vi "sub_psk_symbol_map_gen.vi"(9 "Gray code?":bool=TRUE, 11 "M-PSK":i32=4) -> (1 "index map":u32[](array[numeric]), 3 "symbol map":cdb[](array[numeric]))   [LabVIEW 2014]
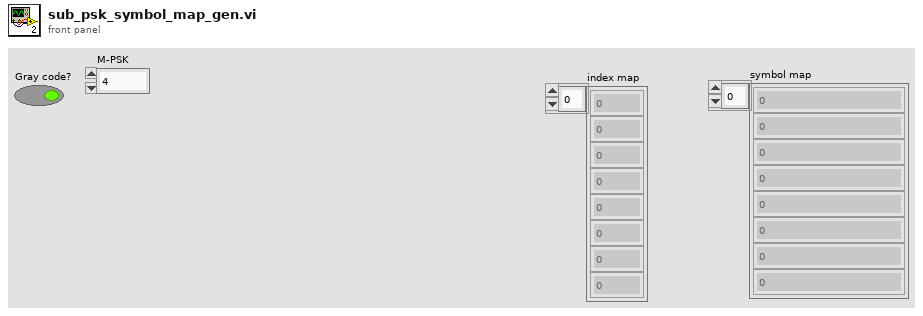
[diagram p1: front panel]
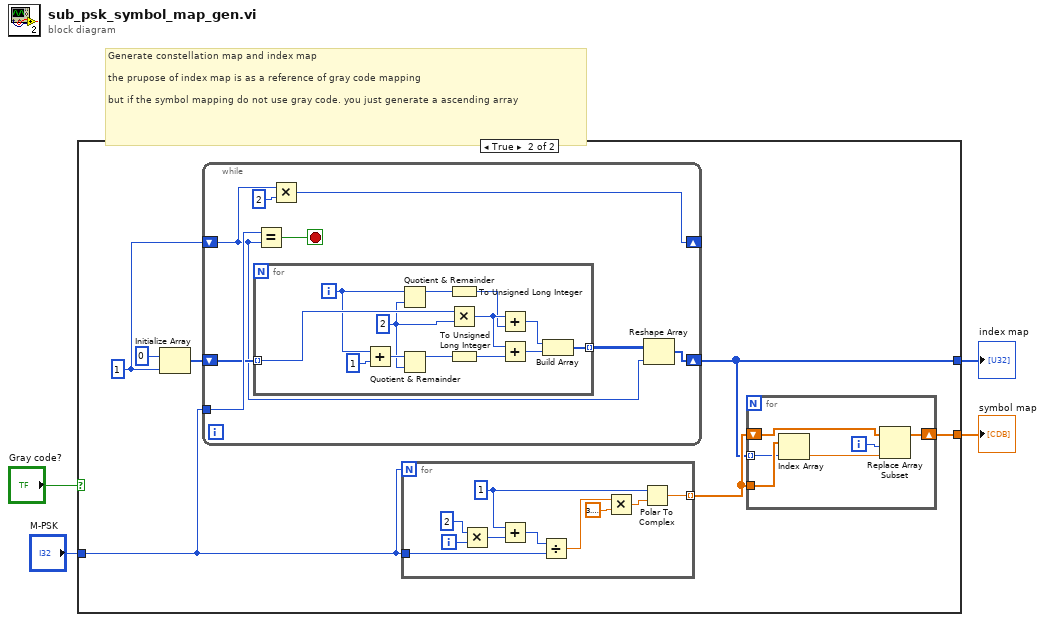
[diagram p0: block diagram]
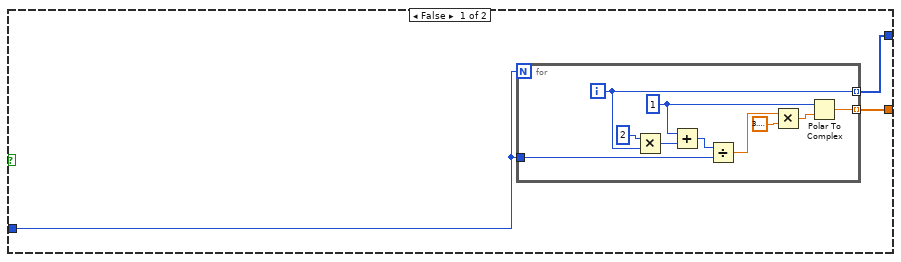
[diagram p2: hidden frame]
diagram:
  # "Generate constellation map and index map\n\nthe prupose of index map is as a reference of gray code mapping\n\nbut if the symbol mapping do not use gray code. you just generate a ascending array"
  n1 = case shown="True" "Gray code?" {
    tunnel: "M-PSK" -> [w6 w24]
    tunnel: [w7 w18] -> w2
    tunnel: [w5 w19] -> w1
    frame False {
      n2 = for {
        N: w6 -> [_]
        tunnel: [w17] -> w7 mode=indexing
        tunnel: w6 -> [w12]
        tunnel: [w8] -> w5 mode=indexing
        i -> [w17]
        w15 = 1
        n3 = Multiply(x=2, y=w17) -> (x*y=w14:i32)
        n4 = Add(x=w15, y=w14) -> (x+y=w13:i32)
        n5 = Divide(x=w13, y=w12) -> (x/y=w11:dbl)
        n6 = Multiply(x=w11, y=3.141592653589793) -> (x*y=w9:dbl)
        n7 = Polar To Complex(1:w9, 2:w15) -> (0:w8:cdb)
      }
    }
    frame True {
      w21 = u32 1
      n8 = Initialize Array(u32 0, w21) -> (w22:u32[])
      n9 = while {
        tunnel: w24 -> [w36]
        shift-right: [w38] -> _
        shift-left: w21 -> [w32]
        shift-right: [w31] -> w18
        shift-left: w22 -> [w34]
        stop <- w35 stop-if-true
        n10 = for {
          tunnel: w34 -> [w51] mode=indexing
          tunnel: [w41] -> w33 mode=indexing
          i -> [w50]
          w47 = u32 2
          n11 = Add(x=w50, y=u32 1) -> (x+y=w48:u32)
          n12 = Quotient & Remainder(x=w50, y=w47) -> (x-y*floor(x/y)=w40:u32)  [unwired: 1 out]
          n13 = Quotient & Remainder(x=w48, y=w47) -> (x-y*floor(x/y)=w39:u32)  [unwired: 1 out]
          n14 = To Unsigned Long Integer(number=w40) -> (unsigned 32bit integer=w43:u32)
          n15 = Multiply(x=w51, y=w47) -> (x*y=w44:u32)
          n16 = To Unsigned Long Integer(number=w39) -> (unsigned 32bit integer=w42:u32)
          n17 = Add(x=w44, y=w43) -> (x+y=w46:u32)
          n18 = Add(x=w44, y=w42) -> (x+y=w45:u32)
          n19 = Build Array(w46, w45) -> (w41:u32[])
        }
        n20 = Equal?(x=w36, y=w32) -> (x = y?=w35:bool)
        n21 = Multiply(x=w32, y=u32 2) -> (x*y=w38:u32)
        n22 = Reshape Array(w33, w32) -> (w31:u32[])
      }
      n23 = for {
        N: w24 -> [_]
        tunnel: w24 -> [w56]
        tunnel: [w52] -> w20 mode=indexing
        i -> [w61]
        w59 = 1
        n24 = Multiply(x=2, y=w61) -> (x*y=w58:i32)
        n25 = Add(x=w59, y=w58) -> (x+y=w57:i32)
        n26 = Divide(x=w57, y=w56) -> (x/y=w55:dbl)
        n27 = Multiply(x=w55, y=3.141592653589793) -> (x*y=w53:dbl)
        n28 = Polar To Complex(1:w53, 2:w59) -> (0:w52:cdb)
      }
      n29 = for {
        tunnel: w20 -> [w30]
        tunnel: w18 -> [w29] mode=indexing
        shift-right: [w25] -> w19
        shift-left: w20 -> [w28]
        i -> [w27]
        n30 = Index Array(array=w30, index=w29) -> (element=w26:cdb)
        n31 = Replace Array Subset(array=w28, new element=w26, index=w27) -> (w25:cdb[])
      }
    }
  }
  "symbol map" <- w1
  "index map" <- w2
